vi "Filter_Table_Test.vi"() -> ()   [LabVIEW 2025, in "CAN-LIN Raw Bus Capture UI.lvlib" / "Table_Filtering.lvlib"]
uses:
  Table_Filtering.lvlib
  <vilib>/Utility/miscctls.llb/LVRowAndColumnUnsignedTypeDef.ctl
panel:
  out "Error Out":errorcluster
  in  "Filter String":string="Protocol == UDP AND Length > 0.7 OR Source == 192.168.1.1"
  in  "Sort by":u16(ring) items=["Packet_Number", "Timestamp", "Source", "Destination", "Protocol", "Length", "Data"]
  in  "Headers":string[](array[string])=["Packet_Number", "Timestamp", "Source", "Destination", "Protocol", "Length", "Data"]
  in  "Pause":bool
  out "Table Control":string[][](table)
  in  "stop":bool
  in  "Visible Columns":bool[](array[boolean])=[TRUE, TRUE, TRUE, TRUE, TRUE, TRUE, TRUE]
  # "The filter expression uses the following syntax:\n\nSets of three arguments separated by logical operators.\nSpaces are used to separate keywords.\nEach set of three arguments follows the pattern: Field, Operator, Value.\nExample: \nProtocol == UDP AND Length > 0.7 OR Source == 192.168.1.1\n\nInvalid inputs include:\n\nStandalone logical operators (e.g., AND, OR)\nTerms by themselves\nArgument sets not equal to three in length\nParentheses\nIf an invalid filter is entered, a warning will be generated."
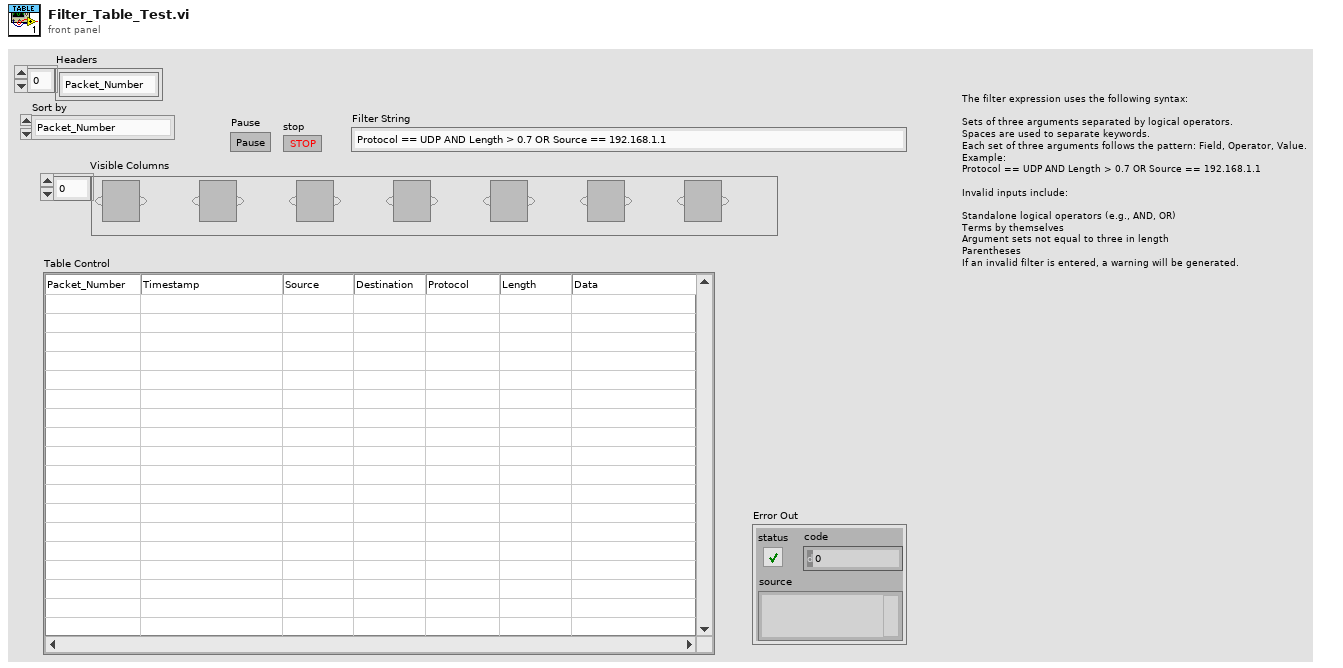
[diagram p1: front panel]
types:
  T1 = typedef "LVRowAndColumnUnsignedTypeDef.ctl" = cluster{"Row":u32, "Column":u32}
  T2 = cluster{"FIELD":string, "OPERATOR":string, "VALUE":string}[]
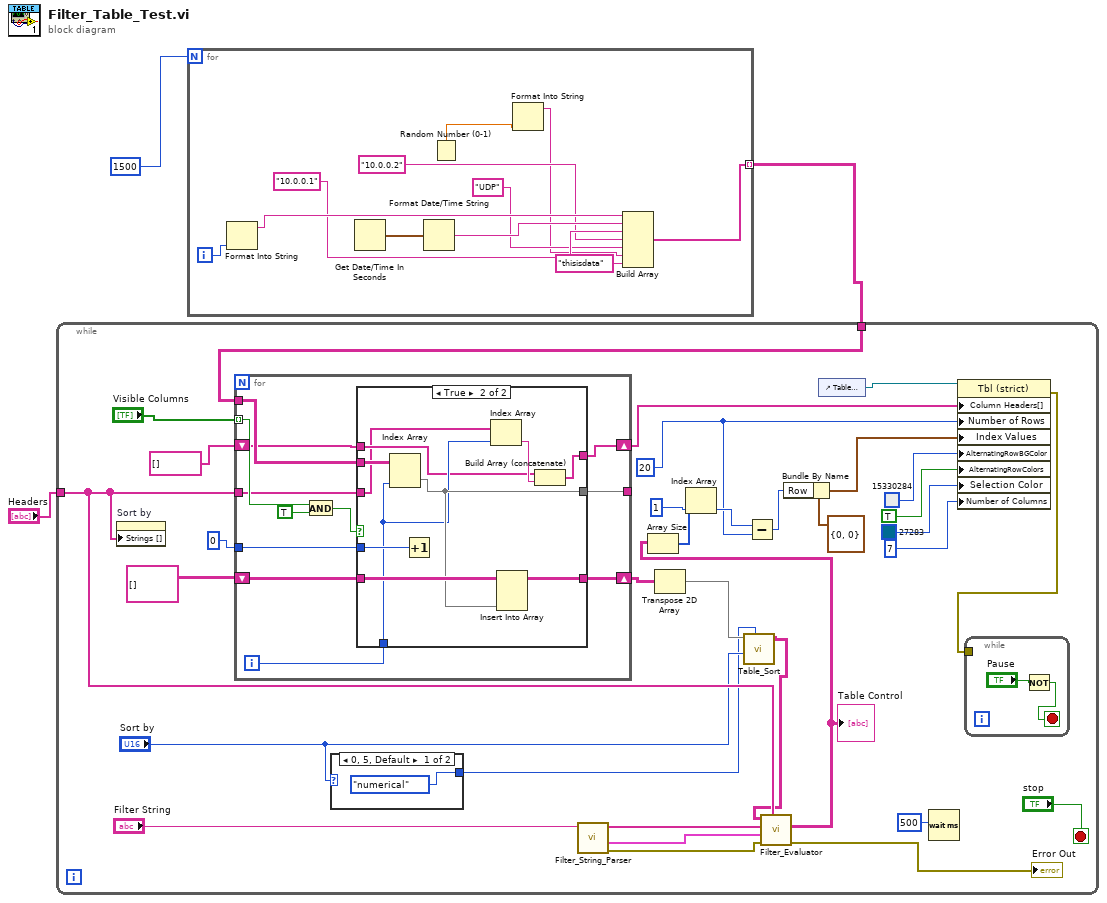
[diagram p0: block diagram]
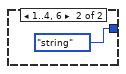
[diagram p2: hidden frame]
diagram:
  n1 = for {
    N: 1500 ("Numeric") -> [_]
    tunnel: [w14] -> w2 mode=indexing
    i -> [w13]
    n2 = Format Into String(w13) -> (resulting string=w12:string)  [unwired: 3 in, 1 out]
    n3 = Get Date/Time In Seconds() -> (seconds since 1Jan1904=w11:timestamp)
    n4 = Format Date/Time String(seconds (now)=w11) -> (date/time string=w10:string)  [unwired: 2 in]
    n5 = Random Number (0-1)() -> (number: 0 to 1=w6:dbl)
    n6 = Format Into String(w6) -> (resulting string=w5:string)  [unwired: 3 in, 1 out]
    n7 = Build Array(w12, w10, "10.0.0.1", "10.0.0.2", "UDP", w5, "thisisdata" ("element")) -> (w14:string[])
  }
  n8 = while {
    tunnel: w2 -> [w47]
    tunnel: "Headers" -> [w22]
    stop <- "stop" stop-if-true
    w38 = u32 20 ("Number of Rows")
    n9 = property on="Sort by" class="Ring (strict)"("Strings []"=w22) -> ()  [unwired: 2 in, 2 out]
    n10 = for {
      tunnel: "Visible Columns" -> [w61] mode=indexing
      tunnel: w47 -> [w63]
      tunnel: [w58] -> _
      shift-right: [w57] -> w42
      shift-left: string[][] [] ("array") -> [w59]
      tunnel: 0 -> [w55]
      shift-right: [w53] -> w44
      shift-left: string[] [] -> [w54]
      tunnel: w22 -> [w52]
      i -> [w62]
      n11 = And(x=w61, y=TRUE) -> (x .and. y?=w56:bool)
      n12 = case shown="True" w56 {
        tunnel: w63 -> [_ w75]
        tunnel: w62 -> [_ w70]
        tunnel: w59 -> [w65 w74]
        tunnel: [_ w73] -> w58
        tunnel: [w65 w72] -> w57
        tunnel: w55 -> [_ w71]
        tunnel: [w64 w69] -> w53
        tunnel: w54 -> [w64 w67]
        tunnel: w52 -> [_ w66]
        frame False {
        }
        frame True {
          n13 = Index Array(array=w75, index (col)=w70) -> (element=w73:string[])  [unwired: 1 in]
          n14 = Increment(x=w71) -> ()  [unwired: 1 out]
          n15 = Index Array(array=w66, index=w70) -> (element=w68:string)
          n16 = Insert Into Array(array=w74, new element=w73) -> (w72:string[][])  [unwired: 2 in]
          n17 = Build Array (concatenate)(w67, w68) -> (w69:string[])
        }
      }
    }
    n18 = case shown="0, 5, Default" "Sort by" {
      tunnel: [enum16{"numerical", "string"}."numerical" ("Sort Type") enum16{"numerical", "string"}."string" ("Sort Type")] -> w17
      frame 0, 5, Default {
      }
      frame 1..4, 6 {
      }
    }
    n19 = call "Filter_String_Parser.vi"("Filter String"="Filter String") -> ("error constant"=w16:errorcluster, "Comparators"=w24:T2, "Boolean Connectors"=w23:string[])  [unwired: 8 in]
    n20 = Transpose 2D Array(2D array=w42) -> (transposed array=w20:string[][])
    n21 = call "Table_Sort.vi"("Sort Type"=w17, "Sort by"="Sort by", "Unsorted Data"=w20) -> ("Sorted data"=w19:string[][])  [unwired: 8 in]
    n22 = call "Filter_Evaluator.vi"("Headers"=w22, "Error"=w16, "Comparators"=w24, "Boolean Connectors"=w23, "Prefiltered Data"=w19) -> ("Error Out"=→"Error Out":errorcluster, "Filtered Array"=w21:string[][])  [unwired: 4 in, 1 out]
    "Table Control" <- w21
    n23 = Array Size(array=w21) -> (size(s)=w41:i32[])
    n24 = Index Array(array=w41, index=1) -> (element=w39:i32)
    n25 = Subtract(x=w39, y=w38) -> (x-y=w37:u32)
    n26 = Bundle By Name(cluster=T1 {"Row"=0, "Column"=0} ("Index Values"), "Row"=w37) -> (w36:T1)
    n27 = control-ref of="Table Control"() -> (w28:refnum<vi>)
    n28 = Wait (ms)(milliseconds to wait=u32 500) -> ()  [unwired: 1 out]
    n29 = property on="Property Node" class="Tbl (strict)"(reference=w28, "Column Headers[]"=w44, "Number of Rows"=w38, "Index Values"=w36, "AlternatingRowBGColor"=u32 15330284 ("Alternate Row Background Color"), "AlternatingRowColors"=TRUE ("Alternating Row Colors"), "Selection Color"=u32 27283, "Number of Columns"=u32 7) -> (error out=w29:errorcluster)  [unwired: 1 in, 1 out]
    n30 = while {
      tunnel: w29 -> [_]
      stop <- w50 stop-if-true
      n31 = Not(x="Pause") -> (.not. x?=w50:bool)
    }
  }
